vi "Log To Disk Example.vi"() -> ()   [LabVIEW 2015, in "VC940.lvlib"]
uses:
  VC940.lvlib
panel:
  in  "Log file path":path
  out "Connection":bool
  out "Display":string
  out "Iteration":i32
  in  "Port name":string="COM1"
  in  "Exit":bool
  # "Instructions\n\nConnect VC940 via serial port and enable send by pressing \"SEND\" button \n(second row center button).  \"SEND\" will appear on display. \nEnter correct serial \"Port name\" in contol below. If you are not sure what \nto enter, open Windows device manager and search for Connections node.\n\nEnter filename for log file with \"Log file path\" browse button or just start VI.\nIn this case log file will be generated in same folder location as this VI.\nThe file is named \"Test.csv\". Can be opened with Microsoft Excel directly.\n\nData will be appended to already existing file (or will be created otherwise). \nEach measurement is written to single line.\nLines consist of three - by semicolons separated - parameters\n1. Time stamp, format DD.MM.YY HH:MM:SS\n2. DMM Function\n3. Measured value as floating point number, if invalid \"not a number=NaN\""
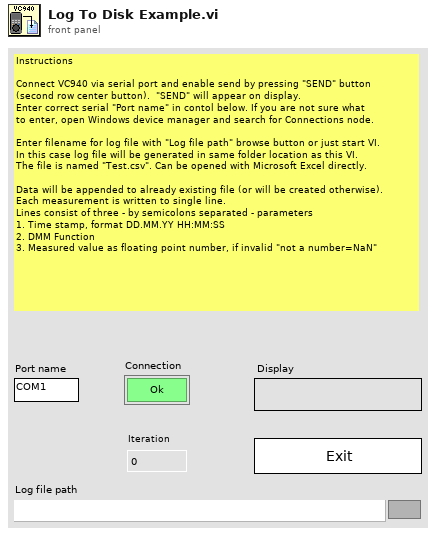
[diagram p1: front panel]
types:
  T1 = enum16{"open", "replace", "create", "open or create", "replace or create", "replace or create with confirmation"}
  T2 = typedef "VC940.lvlib/Function.ctl" = enum8{"mV AC", "V DC", "V AC", "mV DC", "Ohm", "nF", "°C", "µA", "mA", "A", "Ohm Fm", "V Diode", "Hz", "°F", "W", "%4-20mA"}
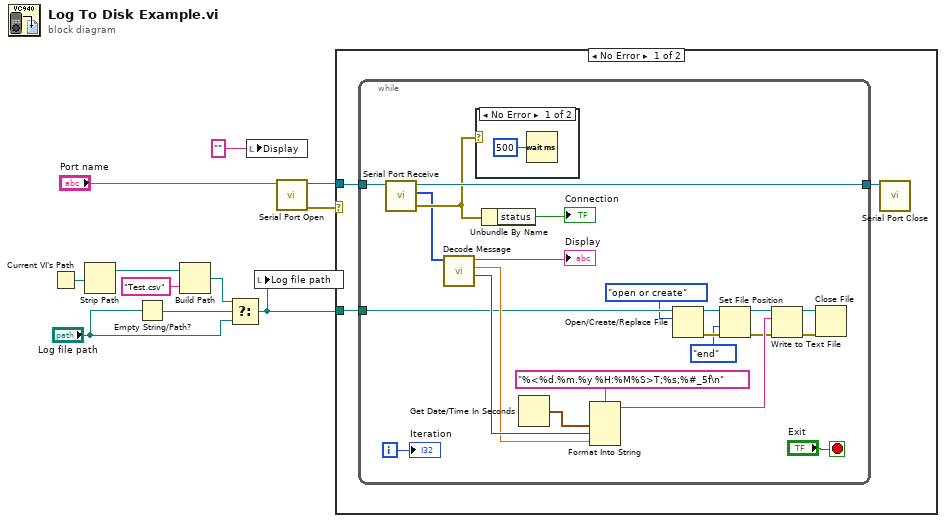
[diagram p0: block diagram]
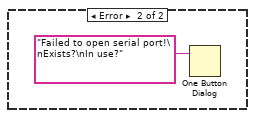
[diagram p3: hidden frame]
diagram:
  n1 = Current VI's Path() -> (path=w7:path)
  n2 = Strip Path(path=w7) -> (stripped path=w6:path)  [unwired: 1 out]
  n3 = Empty String/Path?(string/path="Log file path") -> (empty?=w4:bool)
  n4 = Build Path(base path=w6, name or relative path="Test.csv") -> (appended path=w3:path)
  n5 = Select(t=w3, s=w4, f="Log file path") -> (s? t:f=w1:path)
  n6 = local write "Display"("" ("Data")) -> ()
  n7 = local write "Log file path"(w1) -> ()
  n8 = call "Serial Port Open.vi"("Port name (COM1)"="Port name") -> ("error out"=w8:errorcluster, "Port handle"=w10:refnum<k24>)  [unwired: 9 in]
  n9 = case shown="No Error" w8 {
    tunnel: w10 -> [w14 _]
    tunnel: w1 -> [w12 _]
    frame No Error {
      n10 = while {
        tunnel: w14 -> [w34]
        tunnel: [w33] -> w13
        tunnel: w12 -> [w24]
        i -> [w35]
        stop <- "Exit" stop-if-true
        n11 = call "Serial Port Receive.vi"("Port handle in"=w34) -> ("error out"=w31:errorcluster, "Message"=w29:u8[], "Port handle out"=w33:refnum<k24>)  [unwired: 8 in]
        n12 = call "Decode Message.vi"("Message"=w29) -> ("Function (0..15)"=w26:T2, "Value"=w25:dbl, "Display string"=→"Display":string)  [unwired: 5 in, 3 out]
        n13 = case shown="No Error" w31 {
          frame No Error {
            n14 = Wait (ms)(milliseconds to wait=u32 500) -> ()  [unwired: 1 out]
          }
          frame Error {
          }
        }
        n15 = Unbundle By Name(w31) -> ("status"=→"Connection":bool)
        n16 = Get Date/Time In Seconds() -> (seconds since 1Jan1904=w28:timestamp)
        n17 = Format Into String(format string="%<%d.%m.%y %H:%M%S>T;%s;%#_5f\n", w28, w26, w25) -> (resulting string=w22:string)  [unwired: 2 in, 1 out]
        n18 = Open/Create/Replace File(file path (use dialog)=w24, operation (0:open)=T1."open or create") -> (refnum out=w19:refnum<file>, error out=w17:errorcluster)  [unwired: 4 in, 1 out]
        n19 = Set File Position(refnum=w19, from (0:start)=enum16{"start", "end", "current"}."end", error in=w17) -> (refnum out=w18:refnum<file>, error out=w16:errorcluster)  [unwired: 1 in]
        n20 = Write to Text File(file (use dialog)=w18, text=w22, error in=w16) -> (refnum out=w21:refnum<file>, error out=w20:errorcluster)  [unwired: 1 in, 1 out]
        n21 = Close File(refnum=w21, error in=w20) -> ()  [unwired: 2 out]
        "Iteration" <- w35
      }
      n22 = call "Serial Port Close.vi"("Port handle"=w13) -> ()  [unwired: 10 in, 1 out]
    }
    frame Error {
      n23 = One Button Dialog(message="Failed to open serial port!\nExists?\nIn use?") -> ()  [unwired: 1 in, 1 out]
    }
  }
